vi "MatchImages.vi"(10 "Image2":T1, 11 "Image1":T1) -> (3 "Match":T2)   [LabVIEW 2020, in "2020_20.lvclass"]
uses:
  2020_20.lvclass
  MatchState.ctl
  Image.ctl
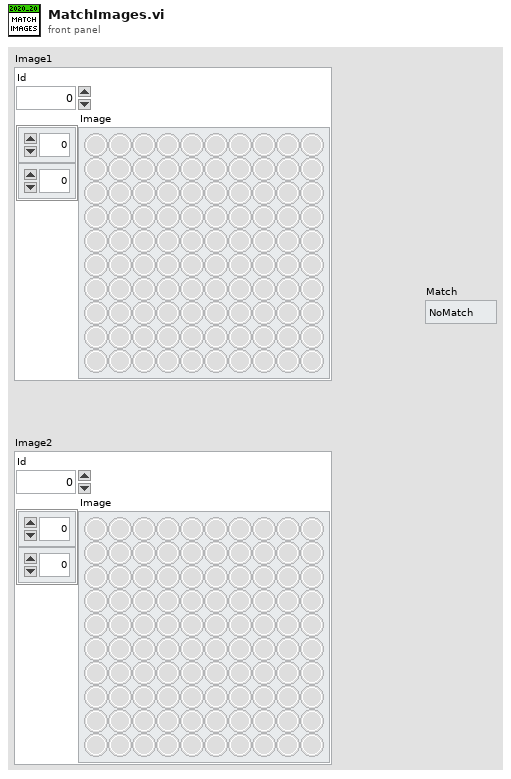
[diagram p1: front panel]
types:
  T1 = typedef "2020_20.lvclass/Image.ctl" = cluster{"Id":i32, "Image":bool[][]}
  T2 = typedef "2020_20.lvclass/MatchState.ctl" = enum16{"NoMatch", "Top", "Right", "Bottom", "Left"}
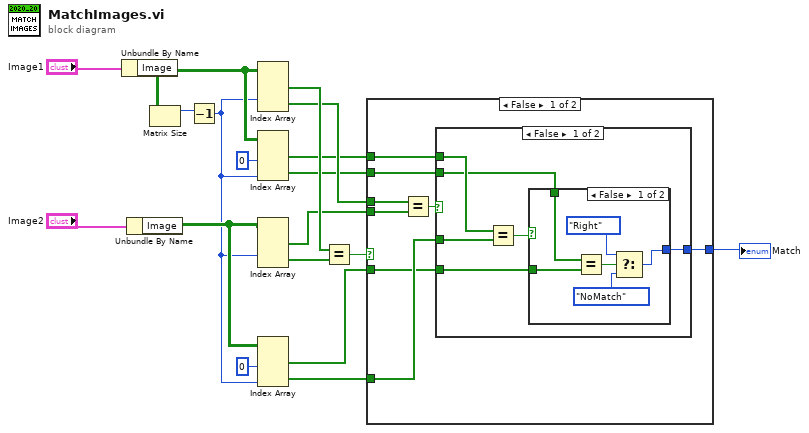
[diagram p0: block diagram]
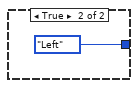
[diagram p2: hidden frame]
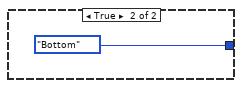
[diagram p3: hidden frame]
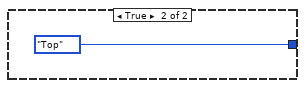
[diagram p4: hidden frame]
diagram:
  n1 = Unbundle By Name("Image1") -> ("Image"=w11:bool[][])
  n2 = Unbundle By Name("Image2") -> ("Image"=w8:bool[][])
  n3 = Matrix Size(0:w11) -> (1:w13:i32)  [unwired: 1 out]
  n4 = Decrement(x=w13) -> (x-1=w7:i32)
  n5 = Index Array(array=w11, index (row) #2=w7) -> (element #1=w16:bool[], element #2=w6:bool[])  [unwired: 3 in]
  n6 = Index Array(array=w11, index (col) #1=0 ("disabled index (col)"), index (col) #2=w7) -> (element #1=w4:bool[], element #2=w2:bool[])  [unwired: 2 in]
  n7 = Index Array(array=w8, index (row) #2=w7) -> (element #1=w5:bool[], element #2=w12:bool[])  [unwired: 3 in]
  n8 = Index Array(array=w8, index (col) #1=0 ("disabled index (col)"), index (col) #2=w7) -> (element #1=w1:bool[], element #2=w3:bool[])  [unwired: 2 in]
  n9 = Equal?(x=w16, y=w12) -> (x = y?=w15:bool)
  n10 = case shown="False" w15 {
    tunnel: [w23 MatchState."Top" ("Match")] -> w14
    tunnel: w6 -> [w26 _]
    tunnel: w5 -> [w25 _]
    tunnel: w4 -> [w22 _]
    tunnel: w3 -> [w21 _]
    tunnel: w2 -> [w20 _]
    tunnel: w1 -> [w19 _]
    frame False {
      n11 = Equal?(x=w26, y=w25) -> (x = y?=w24:bool)
      n12 = case shown="False" w24 {
        tunnel: [w29 MatchState."Bottom" ("Match")] -> w23
        tunnel: w22 -> [w32 _]
        tunnel: w21 -> [w31 _]
        tunnel: w20 -> [w28 _]
        tunnel: w19 -> [w27 _]
        frame False {
          n13 = Equal?(x=w32, y=w31) -> (x = y?=w30:bool)
          n14 = case shown="False" w30 {
            tunnel: [w34 MatchState."Left" ("Match")] -> w29
            tunnel: w28 -> [w38 _]
            tunnel: w27 -> [w37 _]
            frame False {
              n15 = Equal?(x=w38, y=w37) -> (x = y?=w35:bool)
              n16 = Select(t=MatchState."Right" ("Match"), s=w35, f=MatchState."NoMatch" ("Match")) -> (s? t:f=w34:T2)
            }
            frame True {
            }
          }
        }
        frame True {
        }
      }
    }
    frame True {
    }
  }
  "Match" <- w14
